vi "setCost.vi"(8 "error in (no error)":errorcluster, 10 "cost":dbl, 11 "Decaf in":refnum<class "Decaf.lvclass">) -> (0 "error out":errorcluster, 3 "Decaf out":refnum<class "Decaf.lvclass">)   [LabVIEW 2018, in "Decaf.lvclass"]
uses:
  Decaf.lvclass
  Beverage Class/Beverage.lvclass
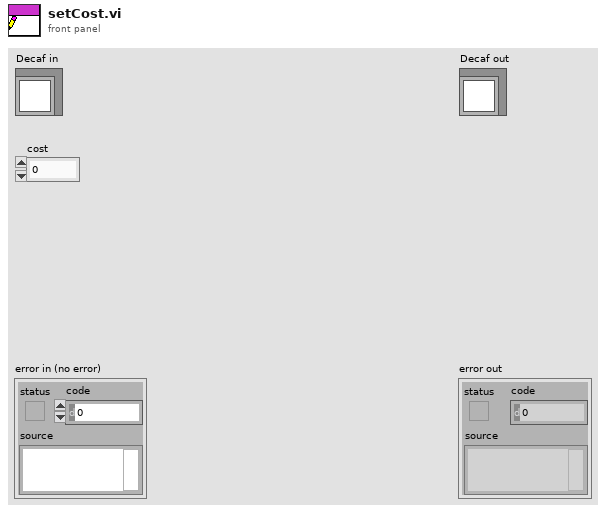
[diagram p1: front panel]
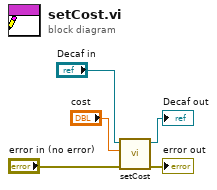
[diagram p0: block diagram]
diagram:
  n1 = call-parent "setCost.vi"("error in (no error)"="error in (no error)", "cost"="cost", "Beverage in"="Decaf in") -> ("error out"=→"error out":errorcluster, "Beverage out"=→"Decaf out":refnum<class "Decaf.lvclass">)  [unwired: 7 in]
